vi "test.vi"() -> ()   [LabVIEW 2020]
uses:
  Includes/DSF Core.lvlibp/Typedefs/DSF Engine Transfer Configuration.ctl
  Includes/DSF Core.lvlibp/Typedefs/Core Transfer Configuration.ctl
  Includes/DSF Core.lvlibp/Typedefs/DSF Settings Info.ctl
  Includes/DSF Core.lvlibp/Typedefs/DSF Engine Channel Configuration.ctl
  Includes/DSF Core.lvlibp/Typedefs/Core Channel Configuration.ctl
  Includes/DSF Core.lvlibp/Typedefs/DSF Data Type.ctl
  Includes/DSF Core.lvlibp/Typedefs/DSF Engine Transfer Group Configuration.ctl
  Includes/DSF Core.lvlibp/Typedefs/Core Group Configuration.ctl
  Includes/DSF Core.lvlibp/Typedefs/DSF Direction.ctl
  Includes/DSF Core.lvlibp/Typedefs/DSF Timing Info.ctl
  Includes/DSF Core.lvlibp/Typedefs/DSF Timeout Behavior.ctl
  Component/Default Buffer Converter/Default Buffer Converter Transfer Settings.ctl
  Includes/DSF Core.lvlibp/Typedefs/DSF Byte Order.ctl
  DSF Configuration API.lvlib
  Includes/DSF Core.lvlibp
  Includes/DSF Core.lvlibp/Classes/Configuration/Core/Channel/Channel Configuration.lvclass
  Includes/DSF Core.lvlibp/Classes/Configuration/Core/Group/Group Configuration.lvclass
  Includes/DSF Core.lvlibp/Classes/Configuration/Core/Transfer/Transfer Configuration.lvclass
panel:
  out "transfer":T1={"core"={"name"="Channel"}, "component settings"=[], "channels"=[]} {"channels"."core"."string offset" format="%d bytes"}
  out "transfer group out":T7={"core"={"name"="Group", "direction"=enum."Tx", "cycle timing"={"priority"=100, "decimation"=1, "offset"=0}, "timeout behavior"=enum."Increment Late Count", "enable conversion"=FALSE}, "component settings"=[], "transfers"=[]} {"transfers"."channels"."core"."string offset" format="%d bytes"}
  out "found? 2":bool
  out "error out 2":errorcluster
  out "removed channel":T4={"core"={"name"="Channel", "units"="V", "engine data type"=enum."DBL", "string data type"=enum."DBL", "string offset"=0}, "component settings"=[]} {"core"."string offset" format="%d bytes"}
  out "transfer out 2":T1={"core"={"name"="Transfer"}, "component settings"=[], "channels"=[]} {"channels"."core"."string offset" format="%d bytes"}
  out "error out":errorcluster
  out "found?":bool
  out "channel":T4={"core"={"name"="Channel", "units"="V", "engine data type"=enum."DBL", "string data type"=enum."DBL", "string offset"=0}, "component settings"=[]} {"core"."string offset" format="%d bytes"}
  out "transfer out":T1={"core"={"name"="Transfer"}, "component settings"=[], "channels"=[]} {"channels"."core"."string offset" format="%d bytes"}
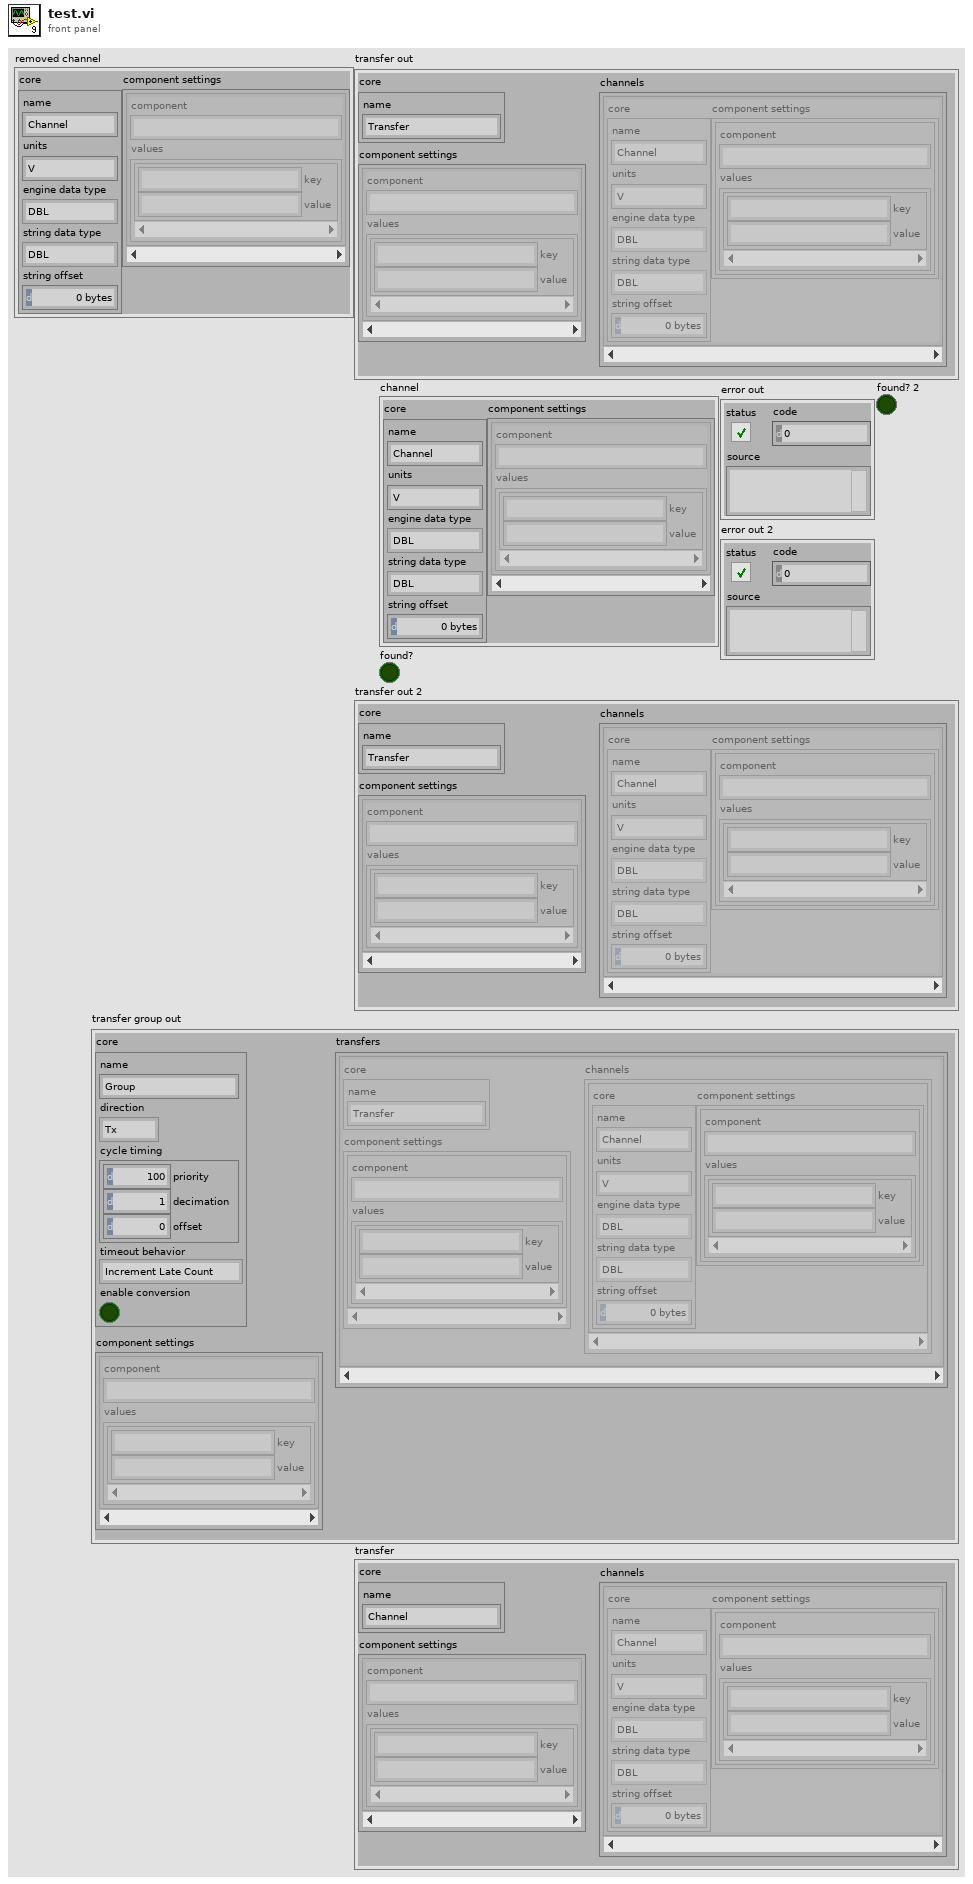
[diagram p1: front panel]
types:
  T1 = typedef "DSF Core.lvlibp/DSF Engine Transfer Configuration.ctl" = cluster{"core":T2, "component settings":T3[], "channels":T4[]}
  T2 = typedef "DSF Core.lvlibp/Transfer Configuration.lvclass/Core Transfer Configuration.ctl" = cluster{"name":string}
  T3 = typedef "DSF Core.lvlibp/DSF Settings Info.ctl" = cluster{"component":string, "values":cluster{"key":string, "value":string}[]}
  T4 = typedef "DSF Core.lvlibp/DSF Engine Channel Configuration.ctl" = cluster{"core":T5, "component settings":T3[]}
  T5 = typedef "DSF Core.lvlibp/Channel Configuration.lvclass/Core Channel Configuration.ctl" = cluster{"name":string, "units":string, "engine data type":T6, "string data type":T6, "string offset":u64}
  T6 = typedef "DSF Core.lvlibp/DSF Data Type.ctl" = enum8{"Bool", "SGL", "DBL", "I8", "I16", "I32", "I64", "U8", "U16", "U32", "U64"}
  T7 = typedef "DSF Core.lvlibp/DSF Engine Transfer Group Configuration.ctl" = cluster{"core":T8, "component settings":T3[], "transfers":T1[]}
  T8 = typedef "DSF Core.lvlibp/Group Configuration.lvclass/Core Group Configuration.ctl" = cluster{"name":string, "direction":T9, "cycle timing":T10, "timeout behavior":T11, "enable conversion":bool}
  T9 = typedef "DSF Core.lvlibp/DSF Direction.ctl" = enum8{"Tx", "Rx"}
  T10 = typedef "DSF Core.lvlibp/DSF Timing Info.ctl" = cluster{"priority":u64, "decimation":u64, "offset":u64}
  T11 = typedef "DSF Core.lvlibp/DSF Timeout Behavior.ctl" = enum8{"Increment Late Count", "Throw Error"}
  T12 = typedef "DSF Configuration API.lvlib/Default Buffer Converter Transfer Settings.ctl" = cluster{"byte order":T13}
  T13 = typedef "DSF Core.lvlibp/DSF Byte Order.ctl" = enum8{"big-endian", "little-endian"}
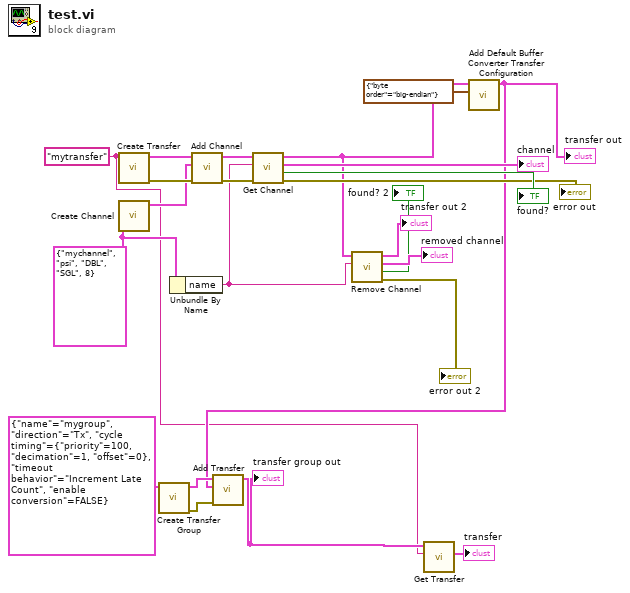
[diagram p0: block diagram]
diagram:
  w19 = T5 {"name"="mychannel", "units"="psi", "engine data type"=enum."DBL", "string data type"=enum."SGL", "string offset"=8} ("channel configuration")
  w2 = "mytransfer" ("name")
  n1 = call "Create Transfer.vi"("name"=w2) -> ("error out"=w22:errorcluster, "transfer"=w23:T1)  [unwired: 9 in]
  n2 = call "Create Channel.vi"("configuration"=w19) -> ("channel out"=w21:T4)  [unwired: 9 in, 1 out]
  n3 = call "Create Transfer Group.vi"("configuration"=T8 {"name"="mygroup", "direction"=enum."Tx", "cycle timing"={"priority"=100, "decimation"=1, "offset"=0}, "timeout behavior"=enum."Increment Late Count", "enable conversion"=FALSE}) -> ("error out"=w7:errorcluster, "transfer group"=w6:T7)  [unwired: 9 in]
  n4 = Unbundle By Name(w19) -> ("name"=w10:string)
  n5 = call "Add Channel.vi"("error in"=w22, "channel"=w21, "transfer"=w23) -> ("error out"=w18:errorcluster, "transfer out"=w20:T1)  [unwired: 7 in]
  n6 = call "Get Channel.vi"("error in"=w18, "channel name"=w10, "transfer"=w20) -> ("error out"=→"error out":errorcluster, "found?"=→"found?":bool, "channel"=→"channel":T4, "transfer out"=w9:T1)  [unwired: 5 in]
  n7 = call "Remove Channel.vi"("channel name"=w10, "transfer"=w9) -> ("error out"=→"error out 2":errorcluster, "found?"=→"found? 2":bool, "removed channel"=→"removed channel":T4, "transfer out"=→"transfer out 2":T1)  [unwired: 6 in]
  n8 = call "Add Default Buffer Converter Transfer Configuration.vi"("transfer settings"=T12 {"byte order"=enum."big-endian"}, "transfer"=w9) -> ("transfer out"=w5:T1)  [unwired: 8 in, 1 out]
  "transfer out" <- w5
  n9 = call "Add Transfer.vi"("error in"=w7, "transfer"=w5, "transfer group"=w6) -> ("transfer group out"=w3:T7)  [unwired: 7 in, 1 out]
  "transfer group out" <- w3
  n10 = call "Get Transfer.vi"("channel name"=w2, "transfer group"=w3) -> ("transfer"=→"transfer":T1)  [unwired: 6 in, 3 out]
